vi "实时数据发送 (子VI).vi"(11 "数值":i32) -> (3 "超时退出":bool)   [LabVIEW 2016, in "数据传输系统.lvlib"]
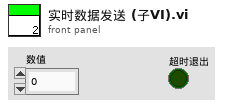
[diagram p1: front panel]
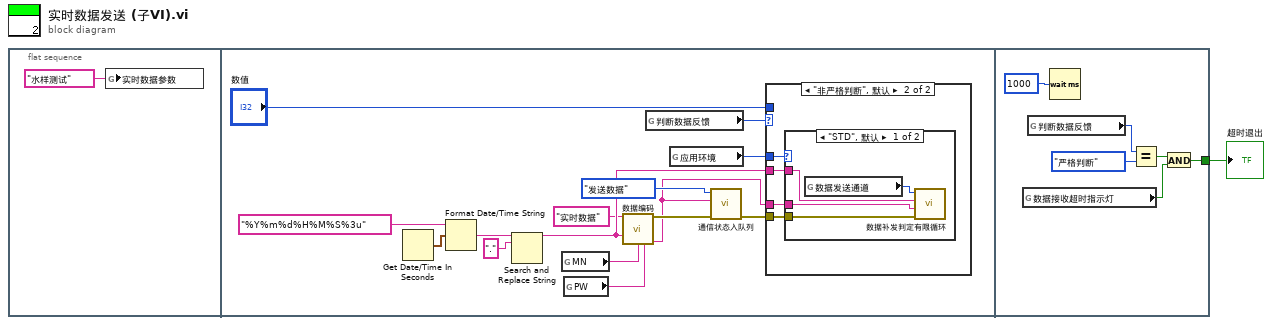
[diagram p0: block diagram]
diagram:
  n1 = flat-sequence {
    tunnel: [w26] -> w1
    frame #0 {
      n2 = global write "全局 实时数据参数.vi" "实时数据参数"("水样测试" ("实时数据参数")) -> ()
    }
    frame #1 {
      n3 = Get Date/Time In Seconds() -> (seconds since 1Jan1904=w15:timestamp)
      n4 = Format Date/Time String(time format string (%c)="%Y%m%d%H%M%S%3u" ("时间格式字符串(%c)"), seconds (now)=w15) -> (date/time string=w14:string)  [unwired: 1 in]
      n5 = Search and Replace String(input string=w14, search string="." ("搜索字符串")) -> (result string=w17:string)  [unwired: 6 in, 3 out]
      n6 = global read "断电保存全局.vi" "MN"() -> (w9:string)
      n7 = global read "断电保存全局.vi" "PW"() -> (w10:string)
      n8 = call "数据编码.vi"("table输入"="实时数据" ("新元素/子数组"), "QN"=w17, "MN"=w9, "PW"=w10) -> ("错误常量"=w8:errorcluster, "通讯包字符串"=w3:string)  [unwired: 10 in]
      n9 = global read "断电保存全局.vi" "判断数据反馈"() -> (w12:enum16{"非严格判断", "严格判断", "不判断"})
      n10 = global read "断电保存全局.vi" "应用环境"() -> (w5:enum16{"STD", "GB212"})
      n11 = call "通信状态入队列.vi"("错误输入（无错误）"=w8, "发送报文"=w3, "枚举"=enum16{"打开连接", "发送数据", "读取数据", "数据处理", "关闭连接"}."发送数据") -> ("错误输出"=w11:errorcluster)  [unwired: 8 in]
      n12 = case shown="\"非严格判断\", 默认" w12 {
        tunnel: w3 -> [_ w21]
        tunnel: w11 -> [_ w20]
        tunnel: "数值" -> [_ _]
        tunnel: w17 -> [_ w19]
        tunnel: w5 -> [_ w18]
        frame "不判断" {
        }
        frame "非严格判断", Default {
          n13 = case shown="\"STD\", 默认" w18 {
            tunnel: w21 -> [w25 _]
            tunnel: w20 -> [w24 _]
            tunnel: w19 -> [w22 _]
            frame "STD", Default {
              n14 = global read "断电保存全局.vi" "数据发送通道"() -> (w23:enum16{"TCP", "VISA"})
              n15 = call "数据补发判定有限循环.vi"("错误输入（无错误）"=w24, "数据输入"=w25, "QN"=w22, "数据发送通道"=w23) -> ()  [unwired: 7 in, 1 out]
            }
            frame "GB212" {
            }
          }
        }
      }
    }
    frame #2 {
      n16 = global read "全局 数据发送重叠.vi" "数据接收超时指示灯"() -> (w27:bool)
      n17 = global read "断电保存全局.vi" "判断数据反馈"() -> (w30:enum16{"非严格判断", "严格判断", "不判断"})
      n18 = Wait (ms)(milliseconds to wait=u32 1000 ("等待时间（毫秒）")) -> ()  [unwired: 1 out]
      n19 = Equal?(x=w30, y=enum16{"非严格判断", "严格判断", "不判断"}."严格判断") -> (x = y?=w28:bool)
      n20 = And(x=w28, y=w27) -> (x .and. y?=w26:bool)
    }
  }
  "超时退出" <- w1
